vi "request.Read id value.vi"(8 "error in (no error)":errorcluster, 11 "Request in":refnum<class "Request.lvclass">) -> (0 "error out":errorcluster, 2 "value":string, 3 "Request out":refnum<class "Request.lvclass">)   [LabVIEW 2020, in "JSON-RPC Lib.lvlib" / "Request.lvclass"]
uses:
  Request.lvclass
  Request.lvclass/Request.ctl
  id/id.Read value.vi
  id/id.lvclass
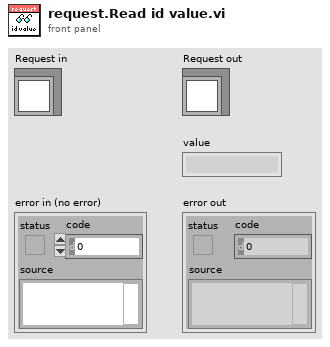
[diagram p1: front panel]
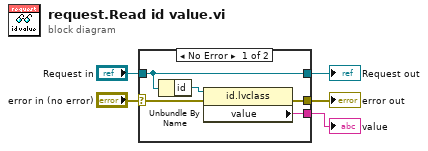
[diagram p0: block diagram]
diagram:
  n1 = case shown="No Error" "error in (no error)" {
    selector: "error in (no error)" -> [w7 w12]
    tunnel: [w6 w12] -> w4
    tunnel: [w10 w11] -> w2
    tunnel: "Request in" -> [w10 w11]
    tunnel: [w8 _] -> w1
    frame No Error {
      n2 = Unbundle By Name(w10) -> ("id"=w9:refnum<class "id.lvclass">)
      n3 = property class="id.lvclass"(reference=w9, error in=w7) -> (error out=w6:errorcluster, "value"=w8:string)  [unwired: 1 out]
    }
    frame Error {
    }
  }
  "error out" <- w4
  "Request out" <- w2
  "value" <- w1
